vi "DAQ Channel Array to ExperimentStateCluster (conflict at 2013-10-03_23-38-54).vi"(8 "Array":T1, 9 "DAQ Channel Array":T3 {"DAQ Channel Array"."Pre Trigger Time" format="%#_6p"; "DAQ Channel Array"."Post Trigger Time" format="%#_6p"; "DAQ Channel Array"."Sample Rate" format="%_3p"}, 11 "Experiment State":T2={"Send Trigger 3"=FALSE, "error"={"status"=FALSE, "code"=0, "source"=""}, "Tasks"={"Fiber15 MP Task"="MyVoltageTask", "Read Slow AI"="", "Fiber Bank DIO"="", "Fiber7 MP Task"="MyVoltageTask", "TaskArray"=[]}, "Channels"={"6133 Channels"=[], "Trigger Source"="", "Edge Type"=10280, "Samples Per Channel"=[], "#Pre-Trigger Samples"=[], "Sample Rate 2.5Ms/s Max"=[]}, "Dev 10 DIO"="", "Dev5"="", "Fiber Triggers 2"=[{"Delay (s)"=2.559999942779541, "Pulse width (s)"=0.009999999776482582, "Active"=TRUE, "Channel Name"="Fiber 8", "counter"="PXI1Slot8/ctr7"}], "MP7"=FALSE, "MP15"=FALSE, "PXI Slot 2"={"PXI Slot 2 Handle"="PXI1Slot2", "source terminal"="GlobalSoftwareTrigger"}, "# of Control DIOs"=0, "Bank DIO Settings"=[], "Purge Duration (s)"=5, "Interlock Override"=FALSE, "Current Raw Voltages, Slot &"=[], "Bank Control"={"Bank Enables"={"Gun1 Enable"=FALSE, "Gun2 Enable"=FALSE, "InnerSol Enable"=FALSE, "OuterSol1 Enable"=FALSE, "Outer2 Enable"=FALSE, "Gun3 Enable"=FALSE}, "Voltages"={"Gun1 Voltage"=0.0, "Gun2 Voltage"=0.0, "Gun3 Voltage"=0.0, "InnerSol Voltage"=0.0, "OuterSol1 Voltage"=0.0, "OuterSol2 Voltage"=0.0}, "Set Points"={"Gun1 Setpoint"=0.0, "Gun2 Setpoint"=0.0, "Gun3 Setpoint"=0.0, "InnerSol Setpoint"=0.0, "OuterSol1 Setpoint"=0.0, "OuterSol2 Setpoint"=0.0}}, "Waveform Data"=[], "Next Shot#"="0", "Slot 7, Last Shot Scaled Voltages"=[], "Data Run Description"="", "Next Shot Data"=["599", "6/18/2009", "4:08PM", "Ziemba", "Bank Testing", "-7.142518", "-8.256295", "-6.893030", "-5.120022", "-0.001235", "-0.001559", "-0.000910", "-0.001235", "-0.001235", "-0.001235", "-0.001235", "0.114909", "-0.000586", "-0.000586", "0.684598", "1.197512"], "Headers"=[], "Html Shot Log View"=FALSE, "ShotLog Headers"=path "", "ShotLog Data"=path "", "Enable Bank Control"=FALSE, "6602  Slot8"={"Slot 8 Trigger Source"="", "Slot 8 Clock Source"="", "Trigger Channel Tasks"=[]}, "6602  Slot 9"={"Slot 9 Clock Source"="", "Slot 9 Trigger Source"="", "Trigger Channel Tasks"=[]}, "Total Sample Time (us)"=[], "Pre-Trigger Time (us)"=[], "Fiber Triggers"=[{"Delay (s)"=2.559999942779541, "Pulse width (s)"=0.009999999776482582, "Active"=TRUE, "Channel Name"="Fiber 8", "counter"="PXI1Slot8/ctr7"}], "System Message"=""} {"Fiber Triggers"."Pulse width (s)" format="%.3p"; "Fiber Triggers"."Delay (s)" format="%.3p"; "Pre-Trigger Time (us)" format="%#_6f"; "Total Sample Time (us)" format="%#_6f"; "Current Raw Voltages, Slot &" format="%0.2f"; "Fiber Triggers 2"."Pulse width (s)" format="%.3p"; "Fiber Triggers 2"."Delay (s)" format="%.3p"; "Channels"."Sample Rate 2.5Ms/s Max" format="%#_3p"; "Channels"."Edge Type" items=["Rising"=10280, "Falling"=10171]}) -> (3 "Experiment State 2":T2={"Send Trigger 3"=FALSE, "error"={"status"=FALSE, "code"=0, "source"=""}, "Tasks"={"Fiber15 MP Task"="MyVoltageTask", "Read Slow AI"="", "Fiber Bank DIO"="", "Fiber7 MP Task"="MyVoltageTask", "TaskArray"=[]}, "Channels"={"6133 Channels"=[], "Trigger Source"="", "Edge Type"=10280, "Samples Per Channel"=[], "#Pre-Trigger Samples"=[], "Sample Rate 2.5Ms/s Max"=[]}, "Dev 10 DIO"="", "Dev5"="", "Fiber Triggers 2"=[{"Delay (s)"=2.559999942779541, "Pulse width (s)"=0.009999999776482582, "Active"=TRUE, "Channel Name"="Fiber 8", "counter"="PXI1Slot8/ctr7"}], "MP7"=FALSE, "MP15"=FALSE, "PXI Slot 2"={"PXI Slot 2 Handle"="PXI1Slot2", "source terminal"="GlobalSoftwareTrigger"}, "# of Control DIOs"=0, "Bank DIO Settings"=[], "Purge Duration (s)"=5, "Interlock Override"=FALSE, "Current Raw Voltages, Slot &"=[], "Bank Control"={"Bank Enables"={"Gun1 Enable"=FALSE, "Gun2 Enable"=FALSE, "InnerSol Enable"=FALSE, "OuterSol1 Enable"=FALSE, "Outer2 Enable"=FALSE, "Gun3 Enable"=FALSE}, "Voltages"={"Gun1 Voltage"=0.0, "Gun2 Voltage"=0.0, "Gun3 Voltage"=0.0, "InnerSol Voltage"=0.0, "OuterSol1 Voltage"=0.0, "OuterSol2 Voltage"=0.0}, "Set Points"={"Gun1 Setpoint"=0.0, "Gun2 Setpoint"=0.0, "Gun3 Setpoint"=0.0, "InnerSol Setpoint"=0.0, "OuterSol1 Setpoint"=0.0, "OuterSol2 Setpoint"=0.0}}, "Waveform Data"=[], "Next Shot#"="0", "Slot 7, Last Shot Scaled Voltages"=[], "Data Run Description"="", "Next Shot Data"=["599", "6/18/2009", "4:08PM", "Ziemba", "Bank Testing", "-7.142518", "-8.256295", "-6.893030", "-5.120022", "-0.001235", "-0.001559", "-0.000910", "-0.001235", "-0.001235", "-0.001235", "-0.001235", "0.114909", "-0.000586", "-0.000586", "0.684598", "1.197512"], "Headers"=[], "Html Shot Log View"=FALSE, "ShotLog Headers"=path "", "ShotLog Data"=path "", "Enable Bank Control"=FALSE, "6602  Slot8"={"Slot 8 Trigger Source"="", "Slot 8 Clock Source"="", "Trigger Channel Tasks"=[]}, "6602  Slot 9"={"Slot 9 Clock Source"="", "Slot 9 Trigger Source"="", "Trigger Channel Tasks"=[]}, "Total Sample Time (us)"=[], "Pre-Trigger Time (us)"=[], "Fiber Triggers"=[{"Delay (s)"=2.559999942779541, "Pulse width (s)"=0.009999999776482582, "Active"=TRUE, "Channel Name"="Fiber 8", "counter"="PXI1Slot8/ctr7"}], "System Message"=""} {"Fiber Triggers"."Pulse width (s)" format="%.3p"; "Fiber Triggers"."Delay (s)" format="%.3p"; "Pre-Trigger Time (us)" format="%#_6f"; "Total Sample Time (us)" format="%#_6f"; "Current Raw Voltages, Slot &" format="%0.2f"; "Fiber Triggers 2"."Pulse width (s)" format="%.3p"; "Fiber Triggers 2"."Delay (s)" format="%.3p"; "Channels"."Sample Rate 2.5Ms/s Max" format="%#_3p"; "Channels"."Edge Type" items=["Rising"=10280, "Falling"=10171]})   [LabVIEW 2012]
doc: "Converts DAQ Channel Array information to Experiment State Cluster format.\n\nOnly takes the first active Trigger from DAQ card array"
uses:
  Controls/DAQ Channel Array.ctl
  Controls/ExperimentStateCluster.ctl
  Controls/Channel Trigger Array.ctl
panel:
  out "Numeric":i32
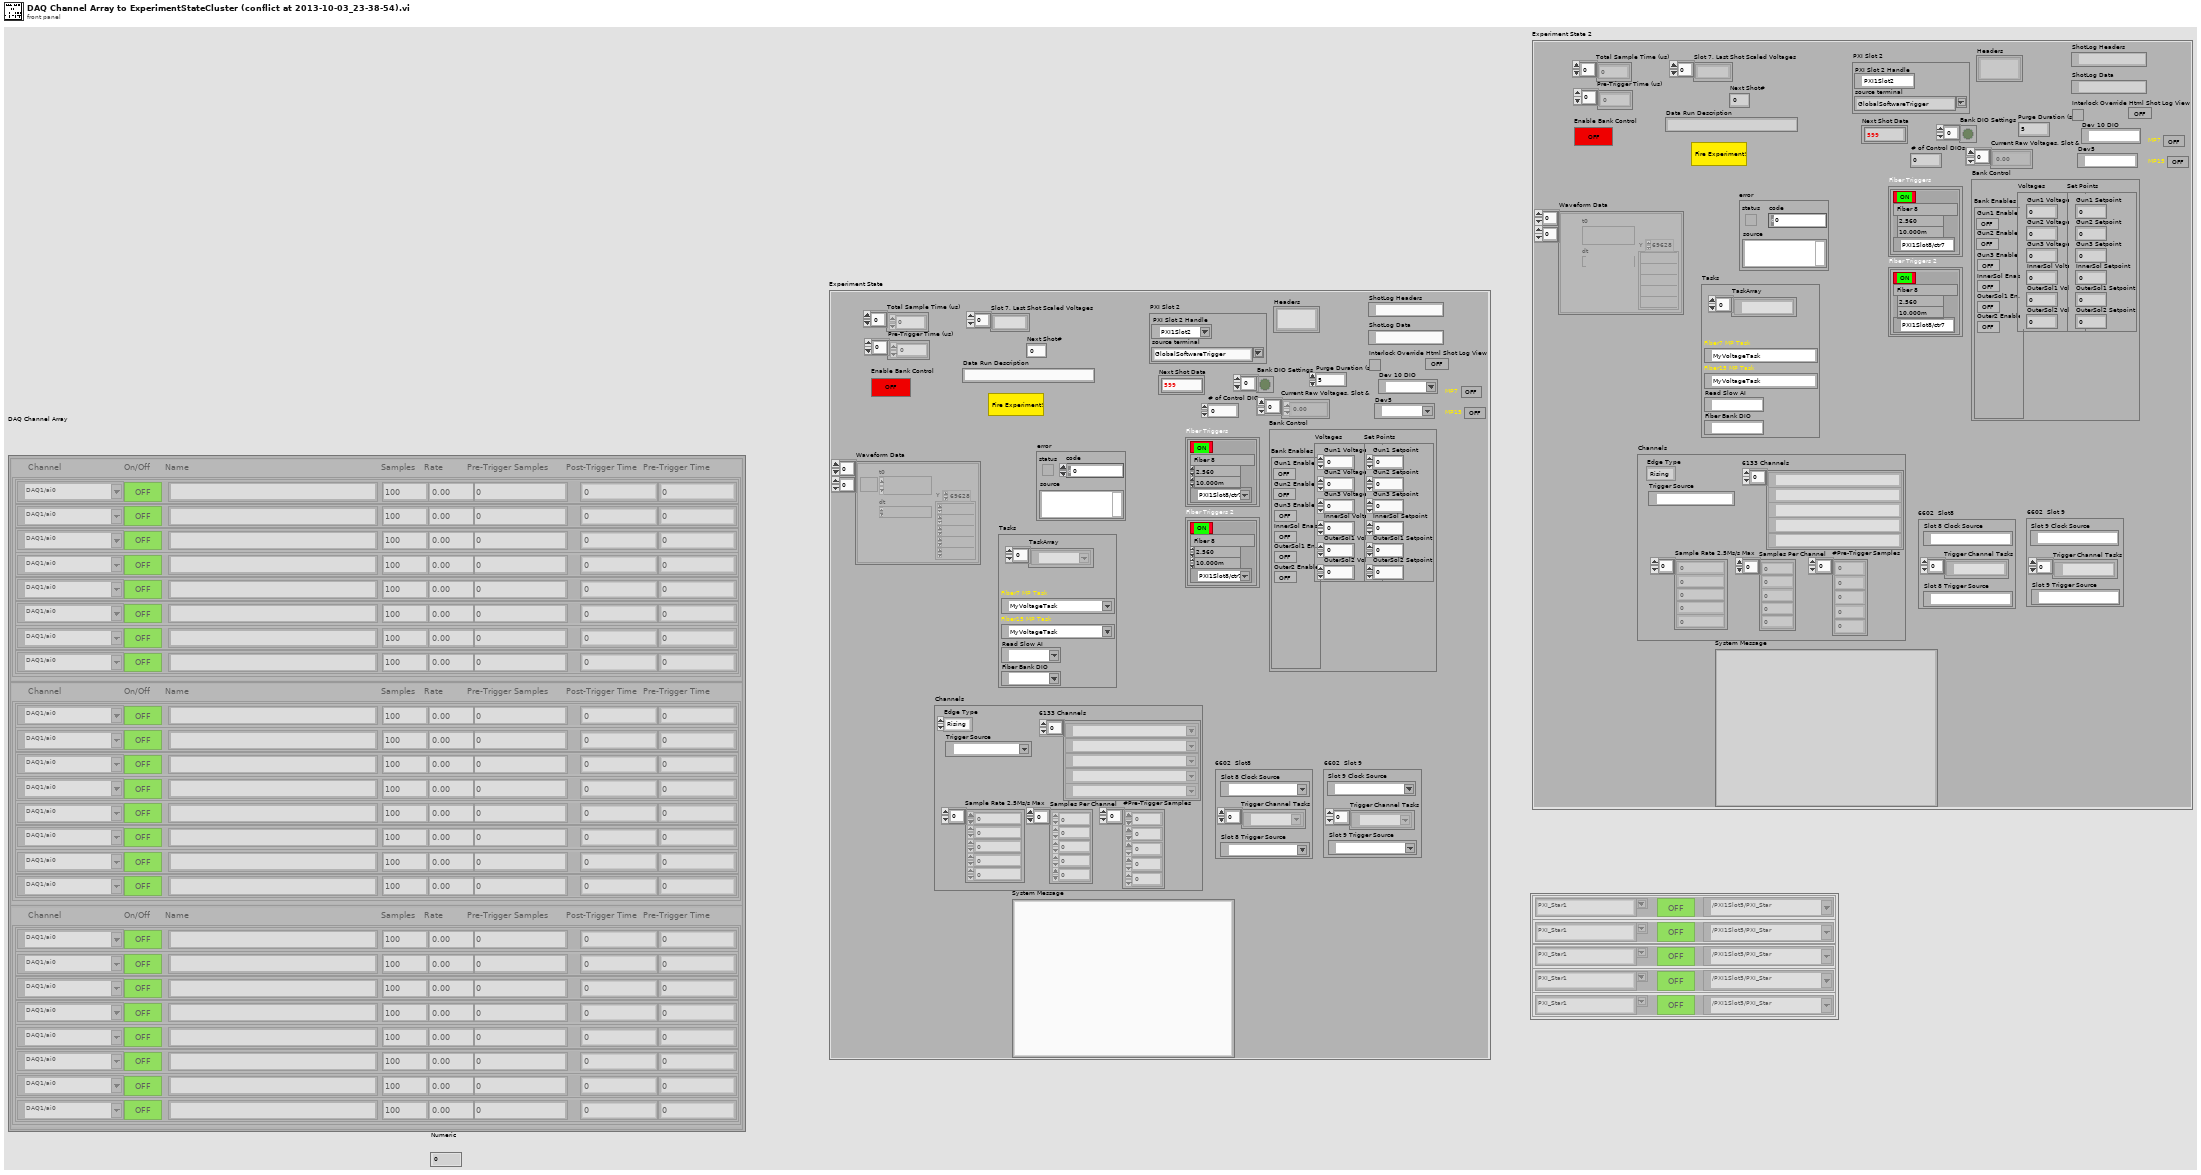
[diagram p1: front panel]
types:
  T1 = typedef "Channel Trigger Array.ctl" = cluster{"Active":bool, "Trigger Source 2":tag, "destination terminal":string}[]
  T2 = typedef "ExperimentStateCluster.ctl" = cluster{"Send Trigger 3":bool, "error":errorcluster, "Tasks":cluster{"Fiber15 MP Task":refnum<k21>, "Read Slow AI":refnum<k21>, "Fiber Bank DIO":refnum<k21>, "Fiber7 MP Task":refnum<k21>, "TaskArray":refnum<k21>[]}, "Channels":cluster{"6133 Channels":tag[], "Trigger Source":tag, "Edge Type":i32, "Samples Per Channel":i32[], "#Pre-Trigger Samples":u32[], "Sample Rate 2.5Ms/s Max":dbl[]}, "Dev 10 DIO":refnum<k21>, "Dev5":refnum<k21>, "Fiber Triggers 2":cluster{"Delay (s)":dbl, "Pulse width (s)":dbl, "Active":bool, "Channel Name":string, "counter":tag}[], "MP7":bool, "MP15":bool, "PXI Slot 2":cluster{"PXI Slot 2 Handle":refnum<k15>, "source terminal":string}, "# of Control DIOs":i32, "Bank DIO Settings":bool[], "Purge Duration (s)":u32, "Interlock Override":bool, "Current Raw Voltages, Slot &":dbl[], "Bank Control":cluster{"Bank Enables":cluster{"Gun1 Enable":bool, "Gun2 Enable":bool, "InnerSol Enable":bool, "OuterSol1 Enable":bool, "Outer2 Enable":bool, "Gun3 Enable":bool}, "Voltages":cluster{"Gun1 Voltage":dbl, "Gun2 Voltage":dbl, "Gun3 Voltage":dbl, "InnerSol Voltage":dbl, "OuterSol1 Voltage":dbl, "OuterSol2 Voltage":dbl}, "Set Points":cluster{"Gun1 Setpoint":dbl, "Gun2 Setpoint":dbl, "Gun3 Setpoint":dbl, "InnerSol Setpoint":dbl, "OuterSol1 Setpoint":dbl, "OuterSol2 Setpoint":dbl}}, "Waveform Data":waveform(dbl)[][], "Next Shot#":string, "Slot 7, Last Shot Scaled Voltages":string[], "Data Run Description":string, "Next Shot Data":string[], "Headers":string[], "Html Shot Log View":bool, "ShotLog Headers":path, "ShotLog Data":path, "Enable Bank Control":bool, "6602  Slot8":cluster{"Slot 8 Trigger Source":tag, "Slot 8 Clock Source":tag, "Trigger Channel Tasks":refnum<k21>[]}, "6602  Slot 9":cluster{"Slot 9 Clock Source":tag, "Slot 9 Trigger Source":tag, "Trigger Channel Tasks":refnum<k21>[]}, "Total Sample Time (us)":dbl[], "Pre-Trigger Time (us)":dbl[], "Fiber Triggers":cluster{"Delay (s)":dbl, "Pulse width (s)":dbl, "Active":bool, "Channel Name":string, "counter":tag}[], "System Message":string}
  T3 = typedef "DAQ Channel Array.ctl" = cluster{"DAQ Channel Array":cluster{"Active":bool, "Channel Name":string, "Sample Rate":dbl, "Samples":i32, "Pre Trigger Samples":i32, "Post Trigger Time":dbl, "Pre Trigger Time":dbl, "Channel":tag}[]}[]
  T4 = cluster{"Active":bool, "Channel Name":string, "Sample Rate":dbl, "Samples":i32, "Pre Trigger Samples":i32, "Post Trigger Time":dbl, "Pre Trigger Time":dbl, "Channel":tag}[]
  T5 = cluster{"Active":bool, "Trigger Source 2":tag, "destination terminal":string}
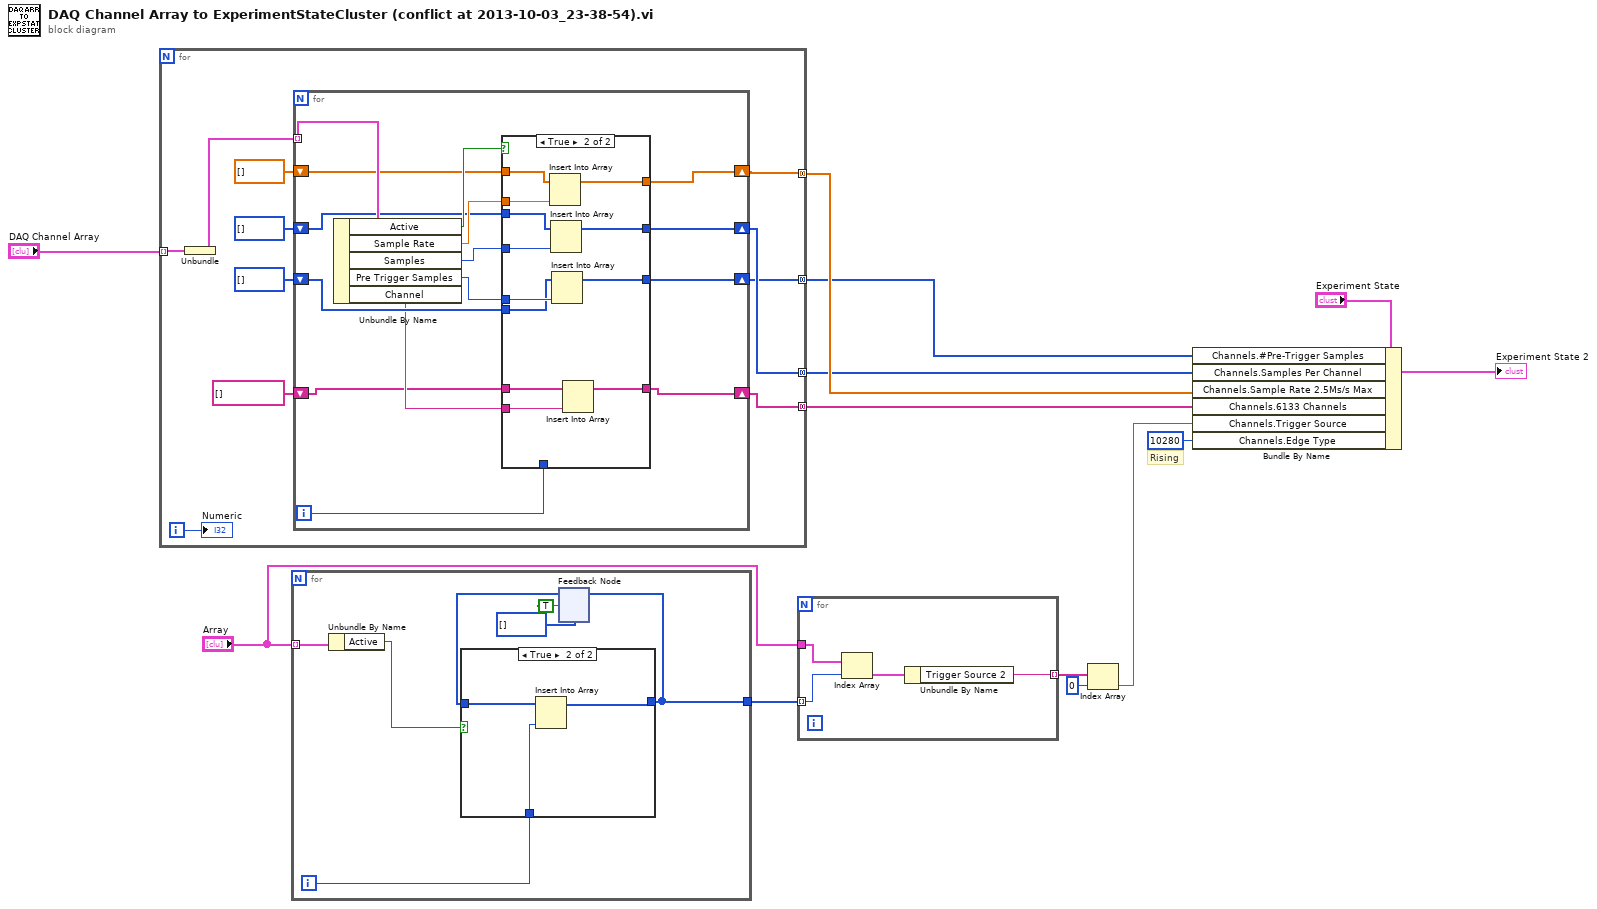
[diagram p0: block diagram]
diagram:
  # "Rising"
  n1 = for {
    tunnel: "DAQ Channel Array" -> [w24] mode=indexing
    tunnel: [w21] -> w4 mode=concatenating
    tunnel: [w16] -> w3 mode=concatenating
    tunnel: [w15] -> w2 mode=concatenating
    tunnel: [w14] -> w1 mode=concatenating
    i -> [w22]
    n2 = Unbundle(w24) -> ("DAQ Channel Array"=w23:T4)
    n3 = for {
      tunnel: w23 -> [w39] mode=indexing
      shift-right: [w35] -> w21
      shift-left: dbl[] [] -> [w34]
      shift-right: [w32] -> w16
      shift-left: i32[] [] -> [w31]
      shift-right: [w29] -> w15
      shift-left: i32[] [] -> [w28]
      shift-right: [w26] -> w14
      shift-left: tag[] [] -> [w25]
      i -> [w37]
      n4 = Unbundle By Name(w39) -> ("Active"=w38:bool, "Sample Rate"=w36:dbl, "Samples"=w33:i32, "Pre Trigger Samples"=w30:i32, "Channel"=w27:tag)
      n5 = case shown="True" w38 {
        tunnel: w37 -> [_ _]
        tunnel: w36 -> [_ w55]
        tunnel: [w43 w54] -> w35
        tunnel: w34 -> [w43 w53]
        tunnel: w33 -> [_ w52]
        tunnel: [w42 w51] -> w32
        tunnel: w31 -> [w42 w50]
        tunnel: w30 -> [_ w49]
        tunnel: [w41 w48] -> w29
        tunnel: w28 -> [w41 w47]
        tunnel: w27 -> [_ w46]
        tunnel: [w40 w45] -> w26
        tunnel: w25 -> [w40 w44]
        frame False {
        }
        frame True {
          n6 = Insert Into Array(array=w53, new element=w55) -> (w54:dbl[])  [unwired: 1 in]
          n7 = Insert Into Array(array=w50, new element=w52) -> (w51:i32[])  [unwired: 1 in]
          n8 = Insert Into Array(array=w47, new element=w49) -> (w48:i32[])  [unwired: 1 in]
          n9 = Insert Into Array(array=w44, new element=w46) -> (w45:tag[])  [unwired: 1 in]
        }
      }
    }
    "Numeric" <- w22
  }
  n10 = for {
    tunnel: "Array" -> [w62] mode=indexing
    tunnel: [w56] -> w10
    i -> [w57]
    n11 = Unbundle By Name(w62) -> ("Active"=w61:bool)
    n12 = feedback #1(i32[] []) -> (w58:i32[])
    n13 = case shown="True" w61 {
      tunnel: w58 -> [w63 w65]
      tunnel: [w63 w64] -> w56
      tunnel: w57 -> [_ w66]
      frame False {
      }
      frame True {
        n14 = Insert Into Array(array=w65, new element=w66) -> (w64:i32[])  [unwired: 1 in]
      }
    }
    n15 = feedback-in #1(w56, TRUE) -> ()
  }
  n16 = for {
    tunnel: w10 -> [w70] mode=indexing
    tunnel: "Array" -> [w69]
    tunnel: [w67] -> w8 mode=indexing
    n17 = Index Array(array=w69, index=w70) -> (element=w68:T5)
    n18 = Unbundle By Name(w68) -> ("Trigger Source 2"=w67:tag)
  }
  n19 = Index Array(array=w8, index=0) -> (element=w5:tag)
  n20 = Bundle By Name(cluster="Experiment State", "Channels.#Pre-Trigger Samples"=w2, "Channels.Samples Per Channel"=w3, "Channels.Sample Rate 2.5Ms/s Max"=w4, "Channels.6133 Channels"=w1, "Channels.Trigger Source"=w5, "Channels.Edge Type"=10280) -> (→"Experiment State 2":T2)
